vi "isPrivateURL.vi"(11 "URL":string) -> (2 "private?":bool, 3 "URL (dup)":string)   [LabVIEW 2014, in "TagDB(dev).lvlib"]
doc: "[Covers: REQ_TAGDB_NAME]\n[Covers: REQ_TAGDB_TEMPNAME]"
uses:
  TagDB(dev).lvlib
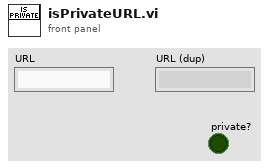
[diagram p1: front panel]
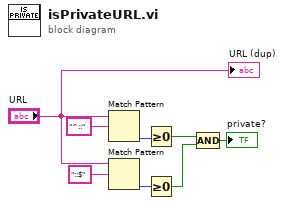
[diagram p0: block diagram]
diagram:
  n1 = Match Pattern(string="URL", regular expression="^::") -> (offset past match=w4:i32)  [unwired: 1 in, 3 out]
  n2 = Match Pattern(string="URL", regular expression="::$") -> (offset past match=w5:i32)  [unwired: 1 in, 3 out]
  n3 = Greater Or Equal To 0?(x=w4) -> (x >= 0?=w6:bool)
  n4 = Greater Or Equal To 0?(x=w5) -> (x >= 0?=w7:bool)
  n5 = Compound Arithmetic op=AND(w6, w7) -> (→"private?":bool)
  "URL (dup)" <- "URL"
